vi "ManageDriversGUI.vi"() -> ()   [LabVIEW 8.6]
panel:
  in  "Refresh":bool
  in  "stop":bool
  in  "drivers":T1(array[cluster])
  # "have to be placed in the driver directory"
  # "start/stop drivers with the running buttton"
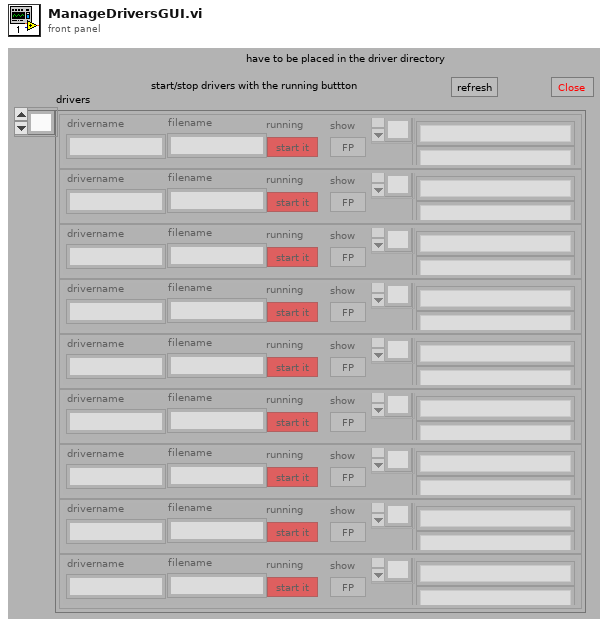
[diagram p1: front panel]
types:
  T1 = cluster{"drivername":string, "filename":string, "running":bool, "variables":string[], "show":bool}[]
  T2 = enum32{"Invalid", "Standard", "Closed", "Hidden", "Minimized", "Maximized"}
  T3 = cluster{"drivername":string, "filename":string, "running":bool, "variables":string[], "show gui":bool}
  T4 = enum16{"None/#Datasets", "Clear", "TagValueOf#", "AddValues", "ReadValue", "ChangeValue", "Get all"}
  T5 = cluster{"drivername":string, "filename":string, "running":bool, "variables":string[], "show":bool}
  T6 = enum32{"Bad", "Idle", "Run top level", "Running"}
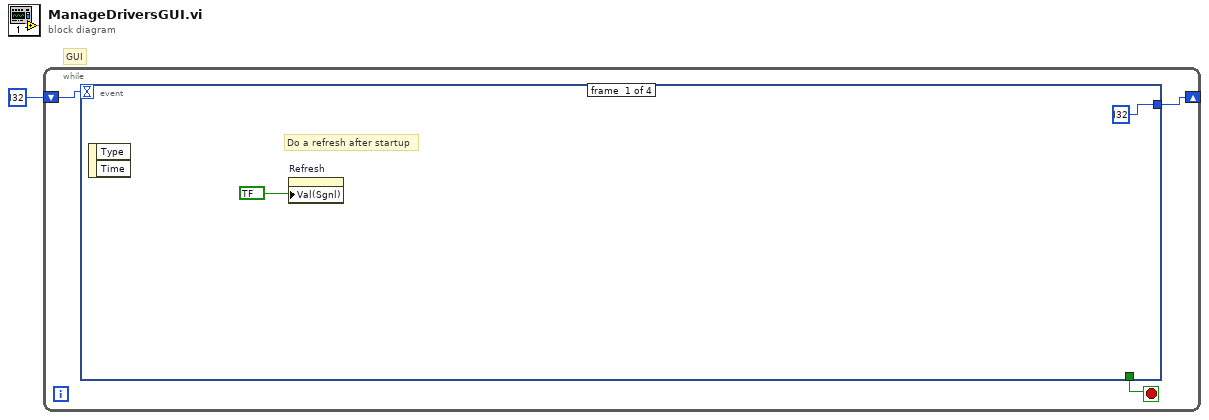
[diagram p0: block diagram]
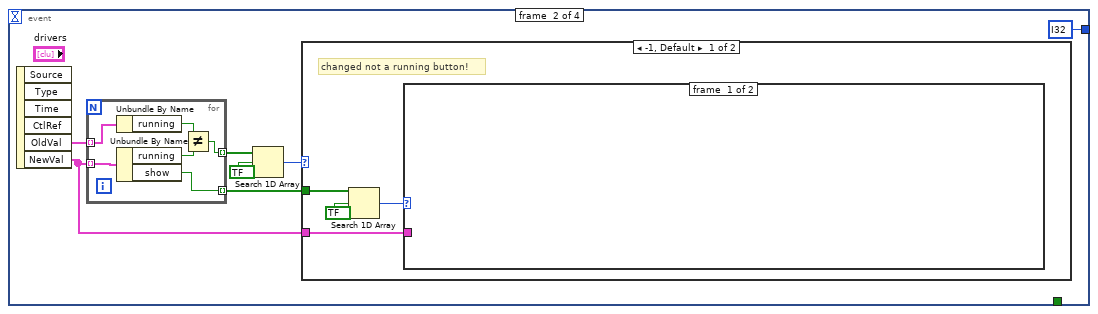
[diagram p2: hidden frame]
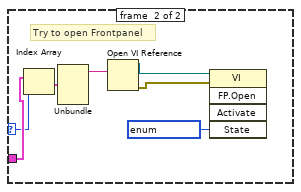
[diagram p3: hidden frame]
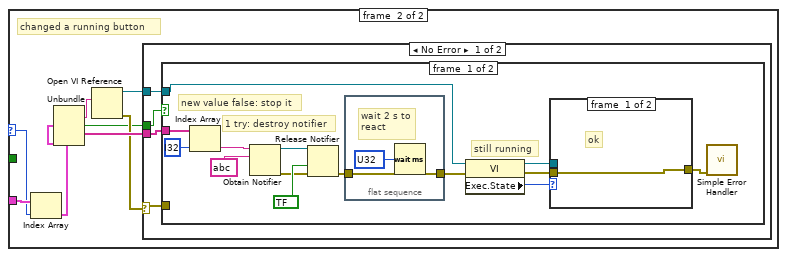
[diagram p4: hidden frame]
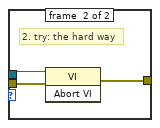
[diagram p5: hidden frame]
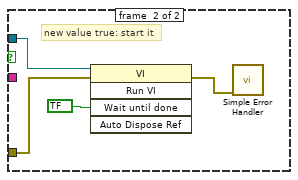
[diagram p6: hidden frame]
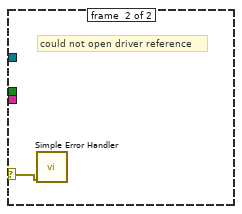
[diagram p7: hidden frame]
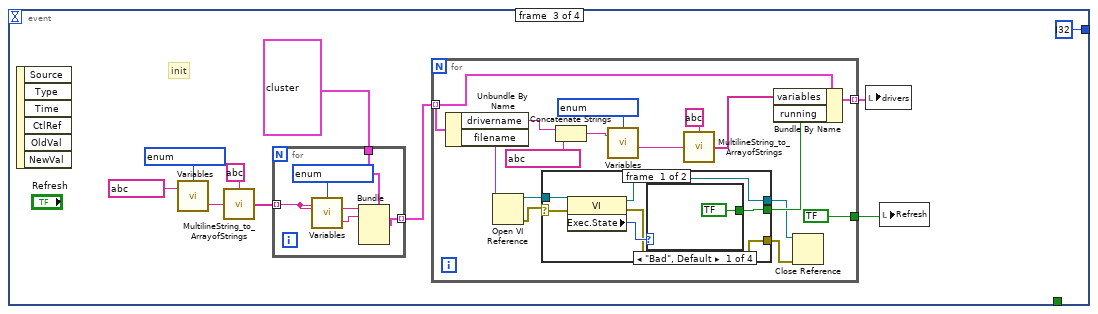
[diagram p8: hidden frame]
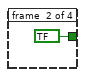
[diagram p9: hidden frame]
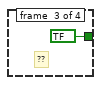
[diagram p10: hidden frame]
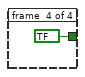
[diagram p11: hidden frame]
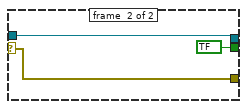
[diagram p12: hidden frame]
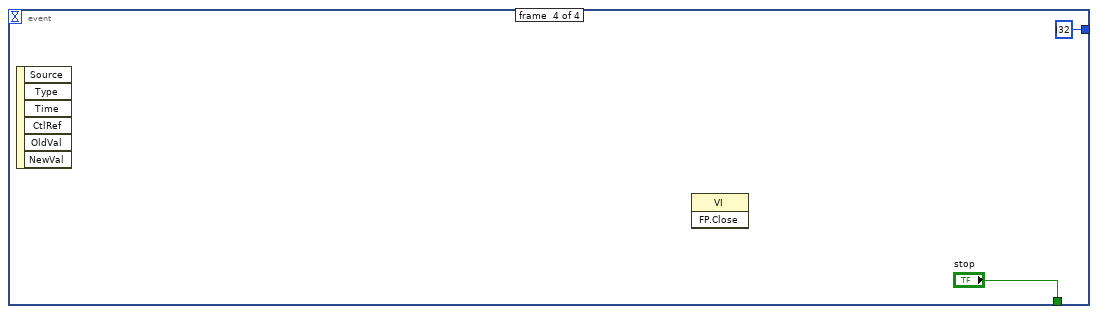
[diagram p13: hidden frame]
diagram:
  # "GUI"
  n1 = while {
    shift-right: [w2] -> _
    shift-left: i32 ? -> [w3]
    stop <- w4 stop-if-true
    n2 = event shown="[2] \"Refresh\": Value Change" {
      selector: _ -> [_ _ _ _]
      dyn-events: _ -> [_ _ _ _]
      timeout: w3 -> [_ _ _ _]
      tunnel: [_ _ _ "stop"] -> w4
      tunnel: [i32 ? i32 ? i32 ? i32 ?] -> w2
      event #0 {
        # "Do a refresh after startup"
        n3 = event-data() -> ()  [unwired: 3 out]
        n4 = property on="Refresh" class="Bool (strict)"("Val(Sgnl)"=bool ?) -> ()  [unwired: 2 in, 2 out]
      }
      event #1 {
        n5 = event-data() -> ("OldVal"=w7:T1, "NewVal"=w10:T1)  [unwired: 5 out]
        n6 = for {
          tunnel: w10 -> [w67] mode=indexing
          tunnel: [w62] -> w13 mode=indexing
          tunnel: [w66] -> w8 mode=indexing
          tunnel: w7 -> [w65] mode=indexing
          n7 = Unbundle By Name(w65) -> ("running"=w64:bool)
          n8 = Unbundle By Name(w67) -> ("running"=w63:bool, "show"=w66:bool)
          n9 = Not Equal?(x=w64, y=w63) -> (x != y?=w62:bool)
        }
        n10 = Search 1D Array(1D array=w13, element=bool ?) -> (index of element=w11:i32)  [unwired: 1 out]
        n11 = case shown="-1, Default" w11 {
          selector: w11 -> [_ w31]
          tunnel: w10 -> [w14 w32]
          tunnel: w8 -> [w16 _]
          frame #0 {
            # "changed not a running button!"
            n12 = Search 1D Array(1D array=w16, element=bool ?) -> (index of element=w15:i32)  [unwired: 1 out]
            n13 = case shown="1.." w15 {
              selector: w15 -> [_ w21]
              tunnel: w14 -> [_ w22]
              frame #0 {
              }
              frame #1 {
                # "Try to open Frontpanel"
                n14 = Index Array(array=w22, index=w21) -> (element=w24:T5)
                n15 = Unbundle(w24) -> ("filename"=w23:string)  [unwired: 4 out]
                n16 = Open VI Reference(vi path=w23) -> (vi reference=w20:refnum<vi>, error out=w18:errorcluster)  [unwired: 1 in, 4 out]
                n17 = invoke class="VI" method="FP.Open"(reference=w20, error in=w18, "State"=T2 ?) -> ()  [unwired: 2 in, 5 out]
              }
            }
          }
          frame #1 {
            # "changed a running button"
            n18 = Index Array(array=w32, index=w31) -> (element=w30:T5)
            n19 = Unbundle(w30) -> ("filename"=w29:string, "running"=w25:bool, "variables"=w27:string[])  [unwired: 2 out]
            n20 = Open VI Reference(vi path=w29) -> (vi reference=w28:refnum<vi>, error out=w26:errorcluster)  [unwired: 1 in, 4 out]
            n21 = case shown="No Error" w26 {
              selector: w26 -> [w33 w61]
              tunnel: w28 -> [w34 _]
              tunnel: w27 -> [w36 _]
              tunnel: w25 -> [w35 _]
              frame #0 {
                n22 = case shown="True" w35 {
                  tunnel: w36 -> [w44 _]
                  tunnel: w34 -> [w41 w58]
                  tunnel: w33 -> [_ w57]
                  frame #0 {
                    # "still running"
                    # "1 try: destroy notifier"
                    # "new value false: stop it"
                    n23 = Index Array(array=w44, index=i32 ?) -> (element=w49:string)
                    n24 = Obtain Notifier(name (unnamed)=w49, notification data type=string ?) -> (notifier out=w47:refnum<notifier>, error out=w45:errorcluster)  [unwired: 2 in, 1 out]
                    n25 = Release Notifier(notifier=w47, force destroy? (F)=bool ?, error in (no error)=w45) -> (error out=w43:errorcluster)  [unwired: 2 out]
                    n26 = flat-sequence {
                      tunnel: w43 -> [w55]
                      tunnel: [w55] -> w42
                      frame #0 {
                        # "wait 2 s to\nreact"
                        n27 = Wait (ms)(milliseconds to wait=u32 ?) -> ()  [unwired: 1 out]
                      }
                    }
                    n28 = property class="VI"(reference=w41, error in=w42) -> (reference out=w39:refnum<vi>, error out=w38:errorcluster, "Exec.State"=w40:T6)
                    n29 = case shown="\"Running\"" w40 {
                      tunnel: w39 -> [_ w54]
                      tunnel: w38 -> [w51 w53]
                      tunnel: [w51 w52] -> w37
                      frame #0 {
                        # "ok"
                      }
                      frame #1 {
                        # "2. try: the hard way"
                        n30 = invoke class="VI" method="Abort VI"(reference=w54, error in=w53) -> (error out=w52:errorcluster)  [unwired: 1 in, 2 out]
                      }
                    }
                    n31 = call <vilib>:"Simple Error Handler.vi"("error in (no error)"=w37) -> ()  [unwired: 2 in, 7 out]
                  }
                  frame #1 {
                    # "new value true: start it"
                    n32 = invoke class="VI" method="Run VI"(reference=w58, error in=w57, "Wait until done"=bool ?) -> (error out=w59:errorcluster)  [unwired: 2 in, 4 out]
                    n33 = call <vilib>:"Simple Error Handler.vi"("error in (no error)"=w59) -> ()  [unwired: 2 in, 7 out]
                  }
                }
              }
              frame #1 {
                # "could not open driver reference"
                n34 = call <vilib>:"Simple Error Handler.vi"("error in (no error)"=w61) -> ()  [unwired: 2 in, 7 out]
              }
            }
          }
        }
      }
      event #2 {
        # "init"
        n35 = event-data() -> ()  [unwired: 7 out]
        n36 = call "Variables.vi"("Tag in"=string ?, "Command"=T4 ?) -> ("value out"=w73:string)  [unwired: 1 in, 2 out]
        n37 = call "MultilineString_to_ArrayofStrings.vi"("String 1"=w73, "NewLineString"=string ?) -> ("String Array"=w75:string[])
        n38 = for {
          tunnel: w75 -> [w80] mode=indexing
          tunnel: T3 ? ("Cluster") -> [w81]
          tunnel: [w78] -> w76 mode=indexing
          n39 = call "Variables.vi"("Tag in"=w80, "Command"=T4 ?) -> ("value out"=w79:string)  [unwired: 1 in, 2 out]
          n40 = Bundle(cluster=w81, "drivername"=w80, "filename"=w79) -> (w78:T3)  [unwired: 3 out]
        }
        n41 = for {
          tunnel: w76 -> [w94] mode=indexing
          tunnel: [w90] -> w77 mode=indexing
          tunnel: [bool ? ("Refresh")] -> w68
          n42 = Unbundle By Name(w94) -> ("drivername"=w98:string, "filename"=w88:string)
          n43 = Open VI Reference(vi path=w88) -> (vi reference=w89:refnum<vi>, error out=w86:errorcluster)  [unwired: 1 in, 4 out]
          n44 = case shown="Error" w86 {
            selector: w86 -> [w101 w109]
            tunnel: w89 -> [w104 w110]
            tunnel: [w102 bool ?] -> w87
            tunnel: [w100 w110] -> w84
            tunnel: [w99 w109] -> w83
            frame #0 {
              n45 = property class="VI"(reference=w104, error in=w101) -> (reference out=w100:refnum<vi>, error out=w99:errorcluster, "Exec.State"=w103:T6)
              n46 = case shown="\"Bad\", Default" w103 {
                tunnel: [bool ? bool ? bool ? bool ?] -> w102
                frame #0 {
                }
                frame #1 {
                }
                frame #2 {
                  # "??"
                }
                frame #3 {
                }
              }
            }
            frame #1 {
            }
          }
          n47 = Concatenate Strings(w98, string ? ("string")) -> (w96:string)
          n48 = call "Variables.vi"("Tag in"=w96, "Command"=T4 ?) -> ("value out"=w92:string)  [unwired: 1 in, 2 out]
          n49 = call "MultilineString_to_ArrayofStrings.vi"("String 1"=w92, "NewLineString"=string ?) -> ("String Array"=w91:string[])
          n50 = Bundle By Name(cluster=w94, "variables"=w91, "running"=w87) -> (w90:T3)
          n51 = Close Reference(reference=w84, error in (no error)=w83) -> ()  [unwired: 1 out]
        }
        n52 = local write "drivers"(w77) -> ()
        n53 = local write "Refresh"(w68) -> ()
      }
      event #3 {
        n54 = event-data() -> ()  [unwired: 7 out]
        n55 = invoke class="VI" method="FP.Close"() -> ()  [unwired: 3 in, 3 out]
      }
    }
  }
